vi "Example Loopback.vi"() -> ()   [LabVIEW 2013]
uses:
  C:/tf/play/labview/Tinkerforge.dll
  Tinkerforge.dll
panel:
  out "message":string
  in  "stop":bool
  in  "uid":string="amb"
  in  "port":i32=4223
  in  "host":string="localhost"
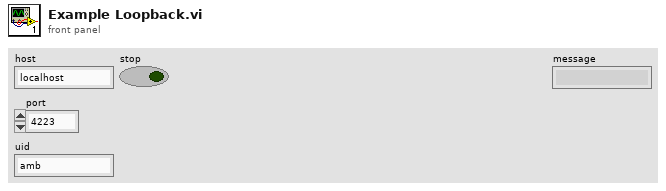
[diagram p1: front panel]
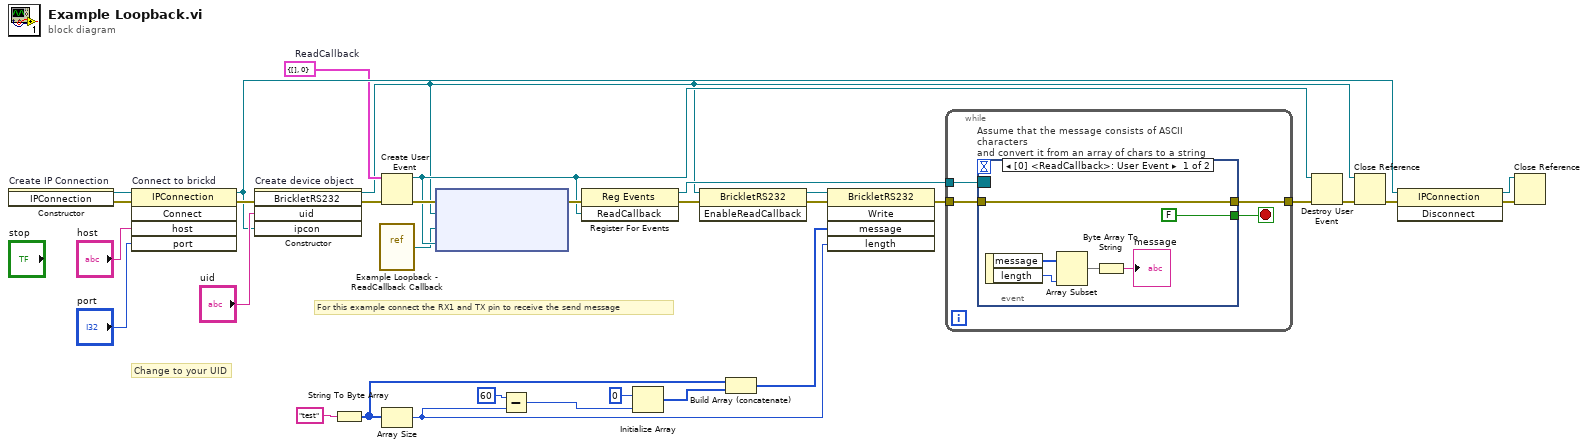
[diagram p0: block diagram]
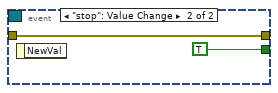
[diagram p2: hidden frame]
diagram:
  w15 = cluster{"message":u16[], "length":u8} {"message"=[], "length"=0}  # ReadCallback
  # "For this example connect the RX1 and TX pin to receive the send message"
  # "Change to your UID"
  n1 = constructor on="Create IP Connection" class="IPConnection"() -> (reference out=w32:refnum<k24>, error out=w17:errorcluster)  [unwired: 3 in, 1 out]
  n2 = invoke on="Connect to brickd" class="IPConnection" method="Connect"(reference=w32, error in=w17, "host"="host", "port"="port") -> (reference out=w25:refnum<k24>, error out=w28:errorcluster)  [unwired: 1 in, 3 out]
  n3 = constructor on="Create device object" class="BrickletRS232"(error in=w28, "uid"="uid", "ipcon"=w25) -> (reference out=w10:refnum<k24>, error out=w11:errorcluster)  [unwired: 2 in, 3 out]
  n4 = String To Byte Array(string="test") -> (unsigned byte array=w3:u8[])
  n5 = vi-ref "Example Loopback - ReadCallback Callback.vi"() -> ("vi reference"=w16:refnum<vi>)
  n6 = Create User Event(user event datatype=w15, error in=w11) -> (user event=w19:refnum<user-event>, error out=w23:errorcluster)
  n7 = Array Size(array=w3) -> (size(s)=w6:i32)
  n8 = node ("Register Event Callback")(w23, w10, w16, w19) -> (w22:errorcluster)  [unwired: 1 in, 1 out]
  n9 = Subtract(x=60, y=w6) -> (x-y=w4:i32)
  n10 = register-events(error in=w22, w19) -> (reference out=w21:refnum<event-registration>, error out=w14:errorcluster)  [unwired: 1 in]
  n11 = Initialize Array(u8 0 ("element"), w4) -> (w2:u8[])
  n12 = invoke class="BrickletRS232" method="EnableReadCallback"(reference=w10, error in=w14) -> (reference out=w9:refnum<k24>, error out=w13:errorcluster)  [unwired: 1 in, 1 out]
  n13 = Build Array (concatenate)(w3, w2) -> (w1:u8[])
  n14 = invoke class="BrickletRS232" method="Write"(reference=w9, error in=w13, "message"=w1, "length"=w6) -> (error out=w12:errorcluster)  [unwired: 1 in, 4 out]
  n15 = while {
    tunnel: w21 -> [w36]
    tunnel: [w35] -> w20
    tunnel: w12 -> [w34]
    stop <- w33 stop-if-true
    n16 = event "Assume that the message consists of ASCII characters\nand convert it from an array of chars to a string" shown="[0] <ReadCallback>: User Event" {
      selector: w36 -> [_ _]
      dyn-events: _ -> [_ _]
      timeout: _ -> [_ _]
      tunnel: [w42 w43] -> w35
      tunnel: w34 -> [w42 w43]
      tunnel: [FALSE TRUE] -> w33
      event User Event {
        n17 = event-data() -> ("message"=w40:u16[], "length"=w39:u8)  [unwired: 1 in]
        n18 = Array Subset(array=w40, length=w39) -> (w38:u16[])  [unwired: 1 in]
        n19 = Byte Array To String(unsigned byte array=w38) -> (string=→"message":string)
      }
      event "stop": Value Change {
        n20 = event-data() -> ()  [unwired: 1 in, 1 out]
      }
    }
  }
  n21 = Destroy User Event(user event=w19, error in=w20) -> (error out=w18:errorcluster)
  n22 = Close Reference(reference=w10, error in (no error)=w18) -> (error out=w27:errorcluster)
  n23 = invoke class="IPConnection" method="Disconnect"(reference=w25, error in=w27) -> (reference out=w24:refnum<k24>, error out=w26:errorcluster)  [unwired: 1 in, 1 out]
  n24 = Close Reference(reference=w24, error in (no error)=w26) -> ()  [unwired: 1 out]
